vi "ReadSubVI.vi"(8 "error in (no error)":errorcluster, 10 "Set Value (Station 01)":string, 11 "Modbus Master in":refnum<class "Modbus Master.lvclass">) -> (0 "error out":errorcluster, 1 "Numeric":dbl, 2 "String":string, 3 "Modbus Master out":refnum<class "Modbus Master.lvclass">)   [LabVIEW 2019]
uses:
  <vilib>/NI/Modbus Library/API/Master/Modbus Master.lvclass
panel:
  out "number":dbl
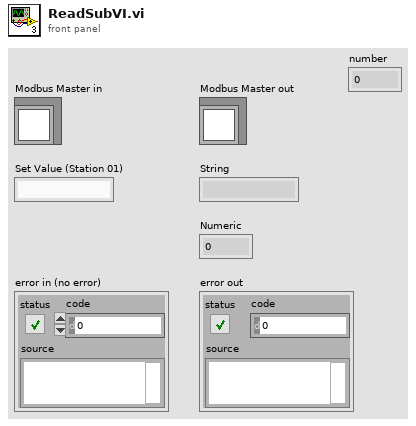
[diagram p1: front panel]
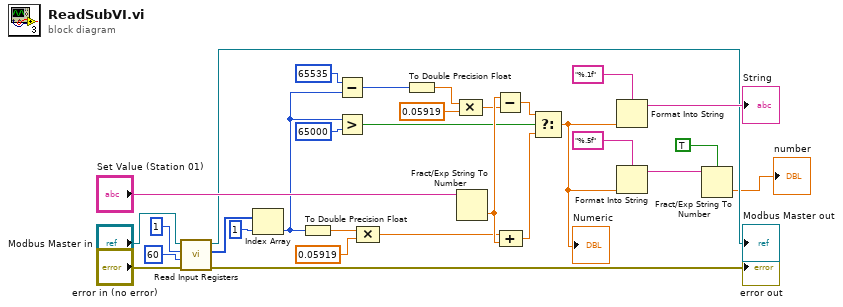
[diagram p0: block diagram]
diagram:
  n1 = call-dynamic "Read Input Registers.vi"("error in"="error in (no error)", "number of inputs"=u16 60 ("number of inputs (Defaut: 60)"), "starting address"=u16 1 ("starting address (Default: 1)"), "Modbus master in"="Modbus Master in") -> ("error out"=→"error out":errorcluster, "register values"=w25:u16[], "Modbus master out"=→"Modbus Master out":refnum<class "Modbus Master.lvclass">)  [unwired: 5 in]
  n2 = Index Array(array=w25, index=1) -> (element=w14:u16)
  n3 = To Double Precision Float(number=w14) -> (double precision float=w17:dbl)
  n4 = Subtract(x=u16 65535 ("y"), y=w14) -> (x-y=w11:u16)
  n5 = Greater?(x=w14, y=u16 65000) -> (0:w7:bool)
  n6 = Compound Arithmetic op=MULTIPLY(w17, 0.05919 ("value")) -> (w23:dbl)
  n7 = To Double Precision Float(number=w11) -> (double precision float=w13:dbl)
  n8 = Fract/Exp String To Number(string="Set Value (Station 01)") -> (number=w26:dbl)  [unwired: 3 in, 1 out]
  n9 = Compound Arithmetic op=MULTIPLY(w13, 0.05919 ("value")) -> (w10:dbl)
  n10 = Subtract(x=w26, y=w10) -> (x-y=w9:dbl)
  n11 = Compound Arithmetic op=ADD(w23, w26) -> (w8:dbl)
  n12 = Select(t=w9, s=w7, f=w8) -> (s? t:f=w6:dbl)
  "Numeric" <- w6
  n13 = Format Into String(format string="%.1f", w6) -> (resulting string=→"String":string)  [unwired: 2 in, 1 out]
  n14 = Format Into String(format string="%.5f", w6) -> (resulting string=w18:string)  [unwired: 2 in, 1 out]
  n15 = Fract/Exp String To Number(use system decimal point (T)=TRUE, string=w18) -> (number=→"number":dbl)  [unwired: 2 in, 1 out]
